vi "niRFUtil MASMT 1D Convolution (CSG).vi"(6 "output size":i32(ring) items=["Full", "Size X", "Compact"], 8 "error in (no error)":errorcluster, 9 "algorithm":i32(ring)=1 items=["Direct", "Frequency Domain"], 10 "Y":csg[](array[numeric]), 11 "X":csg[](array[numeric])) -> (0 "error out":errorcluster, 3 "X * Y":csg[](array[numeric]))   [LabVIEW 2015, in "niRFUtil.lvlib"]
doc: "Computes the convolution of the input sequences <B>X</B> and <B>Y</B>."
uses:
  niRFUtil.lvlib
  Utilities/niRFMASMT_FFT.dll
panel:
  out "FreqWorkH":csg[](array[numeric])
  out "WorkH":csg[](array[numeric])
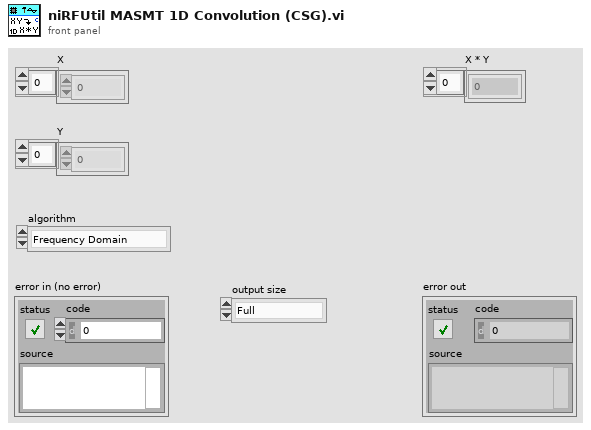
[diagram p1: front panel]
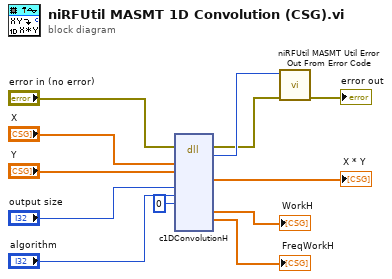
[diagram p0: block diagram]
diagram:
  n1 = dll-call lib="C:/Perforce/semoore-sales/Customers/NATI-3813/Noise Floor/LV Filters/ParallelComplexFilterRFUtil/niRFUtil/MASMT/Utilities/niRFMASMT_FFT.*" fn="c1DConvolutionH"(error in="error in (no error)", "X"="X", "Y"="Y", "size"="output size", "domain"="algorithm", "step"=0) -> (error out=w5:errorcluster, "error"=w7:i32, "X * Y"=→"X * Y":csg[], "WorkH"=→"WorkH":csg[], "FreqWorkH"=→"FreqWorkH":csg[])  [unwired: 12 in, 1 out]
  n2 = call "niRFUtil MASMT Util Error Out From Error Code.vi"("error in (no error)"=w5, "error code"=w7) -> ("error out"=→"error out":errorcluster)  [unwired: 9 in]
